vi "Init Interaction By Reference.vi"(4 "Send events on init? [T]":bool=TRUE, 5 "Pane":refnum<vi>, 6 "Register resize events? [F]":bool, 7 "Sub Panel":refnum<vi>, 8 "error in (no error)":errorcluster, 9 "Resize once? [T]":bool=TRUE, 10 "IObject":refnum<class "IObject.lvclass">) -> (0 "error out":errorcluster, 2 "Object resize event":refnum<event-registration>, 3 "Interaction out":refnum<class "Interaction By Refererence.lvclass">)   [LabVIEW 2013, in "Interaction By Refererence.lvclass"]
uses:
  Interaction By Refererence.lvclass
  IObject.lvclass
  IContainer/Interaction/Interaction.lvclass
  Interaction By Refererence.lvclass/Interaction By Refererence.ctl
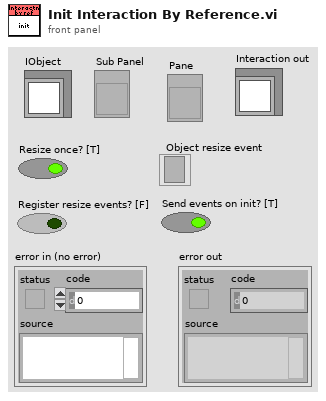
[diagram p1: front panel]
types:
  T1 = typedef "LVRectTypeDef.ctl" = cluster{"Left":i16, "Top":i16, "Right":i16, "Bottom":i16}
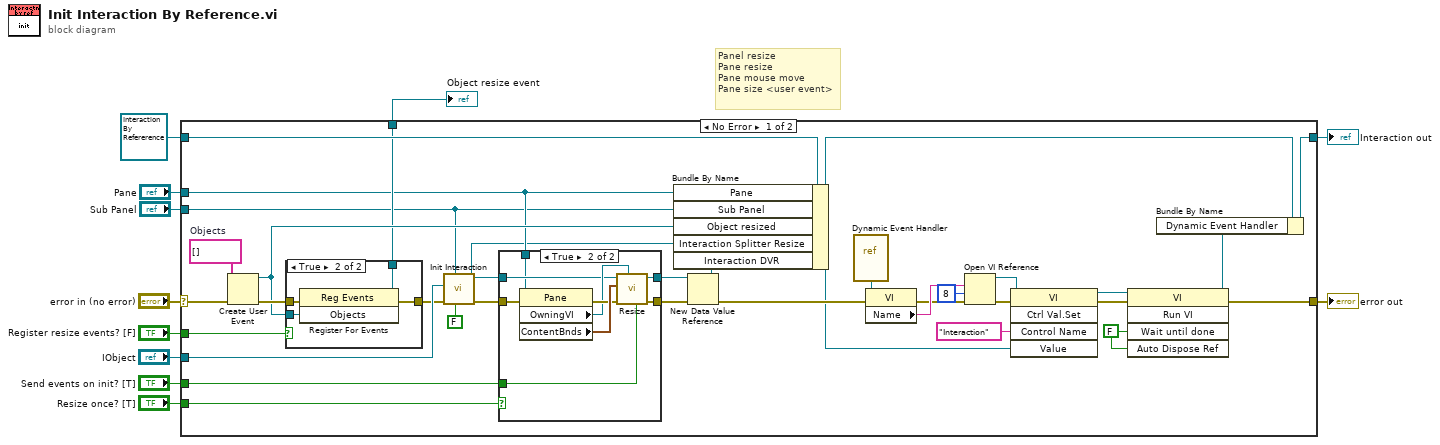
[diagram p0: block diagram]
diagram:
  # "Panel resize\nPane resize\nPane mouse move\nPane size <user event>"
  n1 = case shown="No Error" "error in (no error)" {
    selector: "error in (no error)" -> [w40 w63]
    tunnel: [w22 w63] -> w10
    tunnel: [w15 w62] -> w7
    tunnel: "IObject" -> [w45 _]
    tunnel: "Sub Panel" -> [w27 _]
    tunnel: refnum<class "Interaction By Refererence.lvclass"> refnum ("Interaction out") -> [w44 w62]
    tunnel: "Pane" -> [w28 _]
    tunnel: [w36 _] -> w3
    tunnel: "Register resize events? [F]" -> [w35 _]
    tunnel: "Send events on init? [T]" -> [w32 _]
    tunnel: "Resize once? [T]" -> [w31 _]
    frame No Error {
      w13 = FALSE ("Wait Until Done")
      w34 = string[] []  # Objects
      n2 = Create User Event(user event datatype=w34, error in=w40) -> (user event=w37:refnum<user-event>, error out=w39:errorcluster)
      n3 = case shown="True" w35 {
        tunnel: w39 -> [w57 w61]
        tunnel: [w57 w60] -> w38
        tunnel: w37 -> [_ w59]
        tunnel: [_ w58] -> w36
        frame False {
        }
        frame True {
          n4 = register-events(error in=w61, w59) -> (reference out=w58:refnum<event-registration>, error out=w60:errorcluster)  [unwired: 1 in]
        }
      }
      n5 = call "Init Interaction.vi"("Register for events? [T]"=FALSE, "Sub Panel"=w27, "error in (no error)"=w38, "IObject"=w45) -> ("error out"=w42:errorcluster, "Interaction Splitter Resize"=w12:refnum<user-event>, "Interaction out"=w41:refnum<class "Interaction.lvclass">)  [unwired: 4 in, 1 out]
      n6 = case shown="True" w31 {
        tunnel: [w46 w53] -> w43
        tunnel: w42 -> [w46 w52]
        tunnel: w41 -> [w47 w51]
        tunnel: [w47 w50] -> w29
        tunnel: w28 -> [_ w49]
        tunnel: w32 -> [_ w48]
        frame False {
        }
        frame True {
          n7 = property on="Property Node" class="Pane"(reference=w49, error in=w52) -> (error out=w55:errorcluster, "OwningVI"=w54:refnum<vi>, "ContentBnds"=w56:T1)  [unwired: 1 out]
          n8 = call-dynamic "Resize.vi"("Send events? [T]"=w48, "VI Refnum"=w54, "error in (no error)"=w55, "Bounds"=w56, "MMI Scaling in"=w51) -> ("error out"=w53:errorcluster, "MMI Scaling out"=w50:refnum<class "Interaction.lvclass">)  [unwired: 4 in, 1 out]
        }
      }
      n9 = New Data Value Reference(data value=w29, error in=w43) -> (data value reference=w30:refnum<data-value>, error out=w26:errorcluster)
      n10 = Bundle By Name(cluster=w44, "Pane"=w28, "Sub Panel"=w27, "Object resized"=w37, "Interaction Splitter Resize"=w12, "Interaction DVR"=w30) -> (w16:refnum<class "Interaction By Refererence.lvclass">)
      n11 = vi-ref "Dynamic Event Handler.vi"() -> (w25:refnum<vi>)
      n12 = property class="VI"(reference=w25, error in=w26) -> (error out=w21:errorcluster, "Name"=w24:string)  [unwired: 1 out]
      n13 = Open VI Reference(vi path=w24, options=8, error in (no error)=w21) -> (vi reference=w19:refnum<vi>)  [unwired: 3 in, 1 out]
      n14 = invoke class="VI" method="Ctrl Val.Set"(reference=w19, error in=w21, "Control Name"="Interaction", "Value"=w16) -> (reference out=w18:refnum<vi>, error out=w20:errorcluster)  [unwired: 1 in, 3 out]
      n15 = invoke class="VI" method="Run VI"(reference=w18, error in=w20, "Wait until done"=w13, "Auto Dispose Ref"=w13) -> (reference out=w14:refnum<vi>, error out=w22:errorcluster)  [unwired: 1 in, 3 out]
      n16 = Bundle By Name(cluster=w16, "Dynamic Event Handler"=w14) -> (w15:refnum<class "Interaction By Refererence.lvclass">)
    }
    frame Error {
    }
  }
  "error out" <- w10
  "Interaction out" <- w7
  "Object resize event" <- w3
